vi "Go to Work.vi"(8 "error in (no error)":errorcluster, 11 "Work in":refnum<class "Work.lvclass">) -> (0 "error out":errorcluster, 3 "Chef State out":refnum<class "State Actor.lvclass">)   [LabVIEW 2024, in "Chef State.lvlib" / "Work.lvclass"]
uses:
  Work.lvclass
  Work.lvclass/Work.ctl
  C:/Users/burakkorkmaz/Desktop/PROJE/actor-state-machine/Chef State/Chef State/Chef State.lvclass
  C:/Program Files/National Instruments/LabVIEW 2024/vi.lib/NI/Actors/State Actor/State Actor/State Actor.lvclass
  C:/Program Files/National Instruments/LabVIEW 2024/vi.lib/ActorFramework/Actor/Actor.lvclass
  C:/Users/burakkorkmaz/Desktop/PROJE/actor-state-machine/Chef State/Work/Work.lvclass
  <vilib>/NI/Actors/State Actor/State Actor/State Actor.lvclass
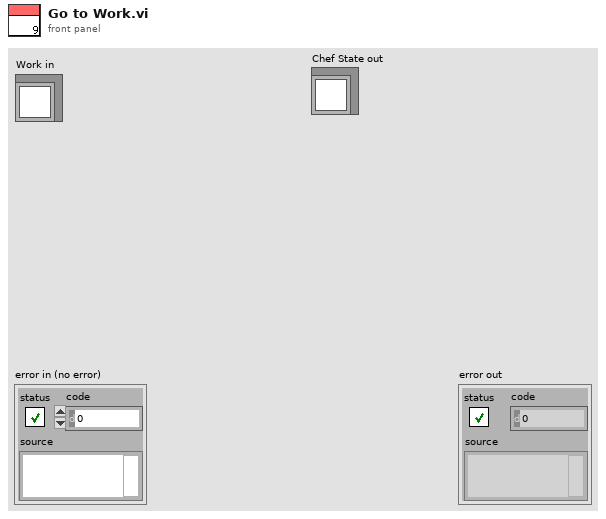
[diagram p1: front panel]
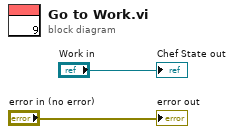
[diagram p0: block diagram]
diagram:
  "error out" <- "error in (no error)"
  "Chef State out" <- "Work in"
